vi "UHR-Fleezers Control (host) - 10.6.vi"() -> ()   [LabVIEW 2011] (continued)
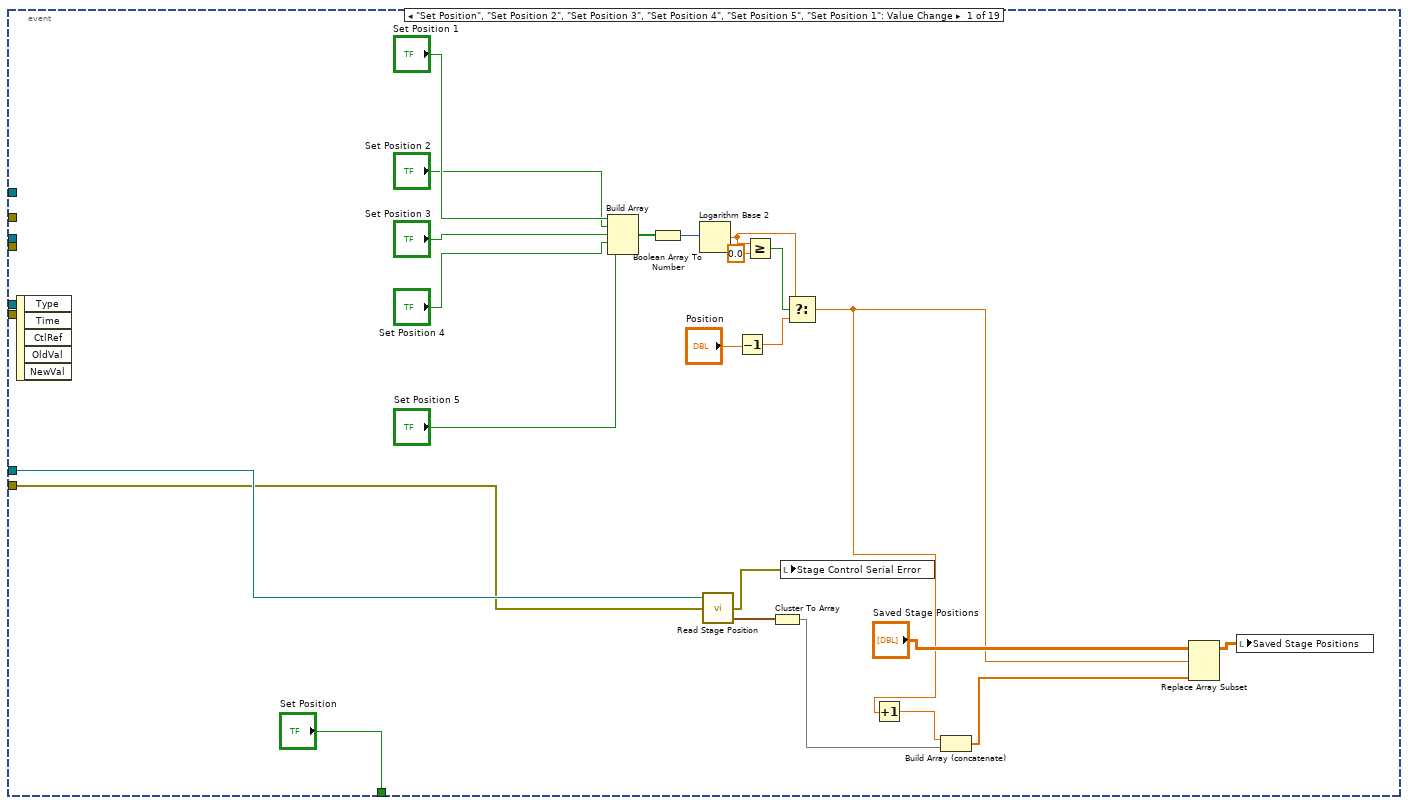
[diagram p2: hidden frame]
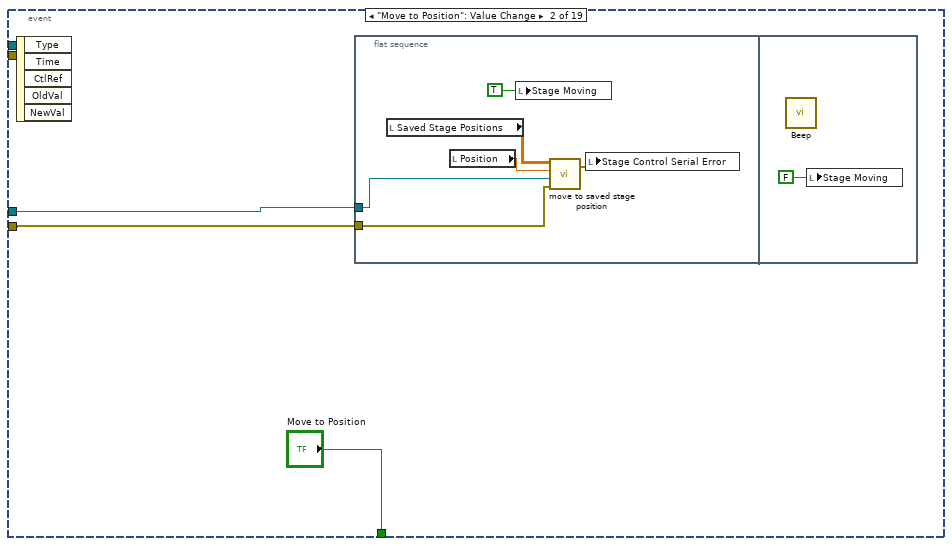
[diagram p3: hidden frame]
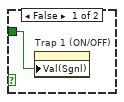
[diagram p5: hidden frame]
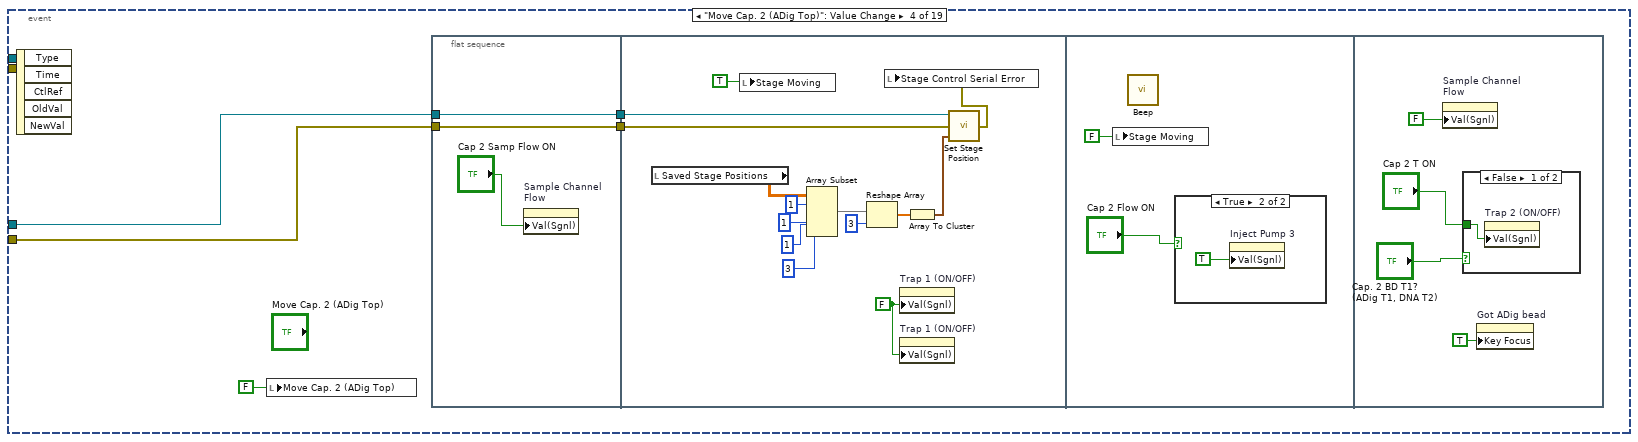
[diagram p6: hidden frame]
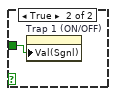
[diagram p8: hidden frame]
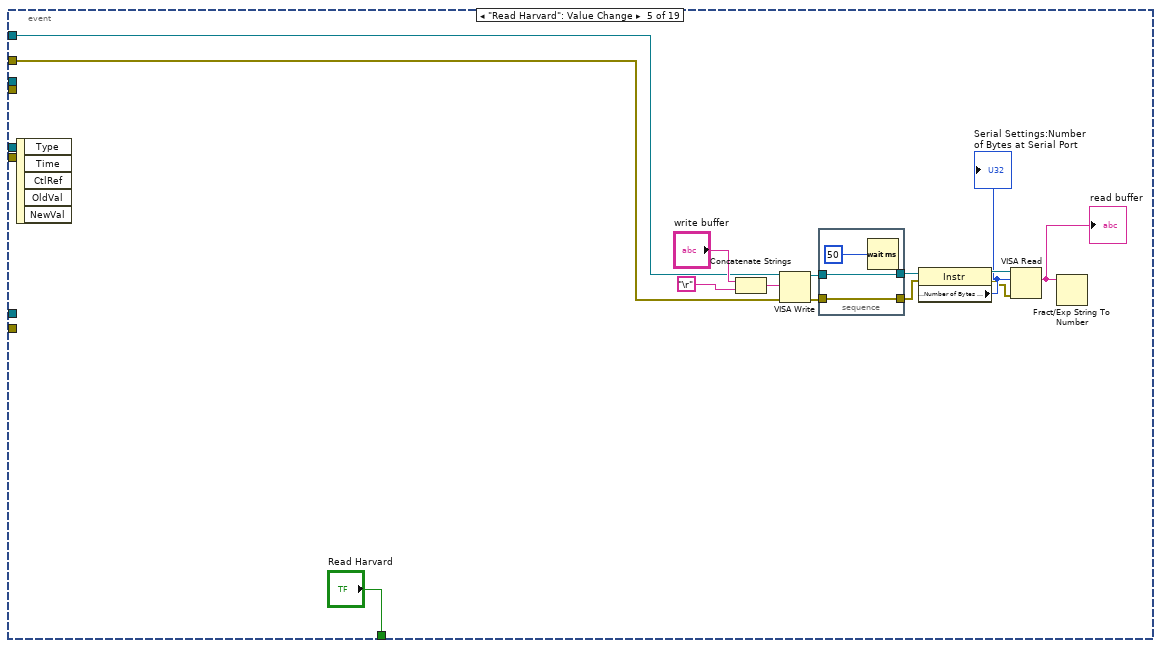
[diagram p9: hidden frame]
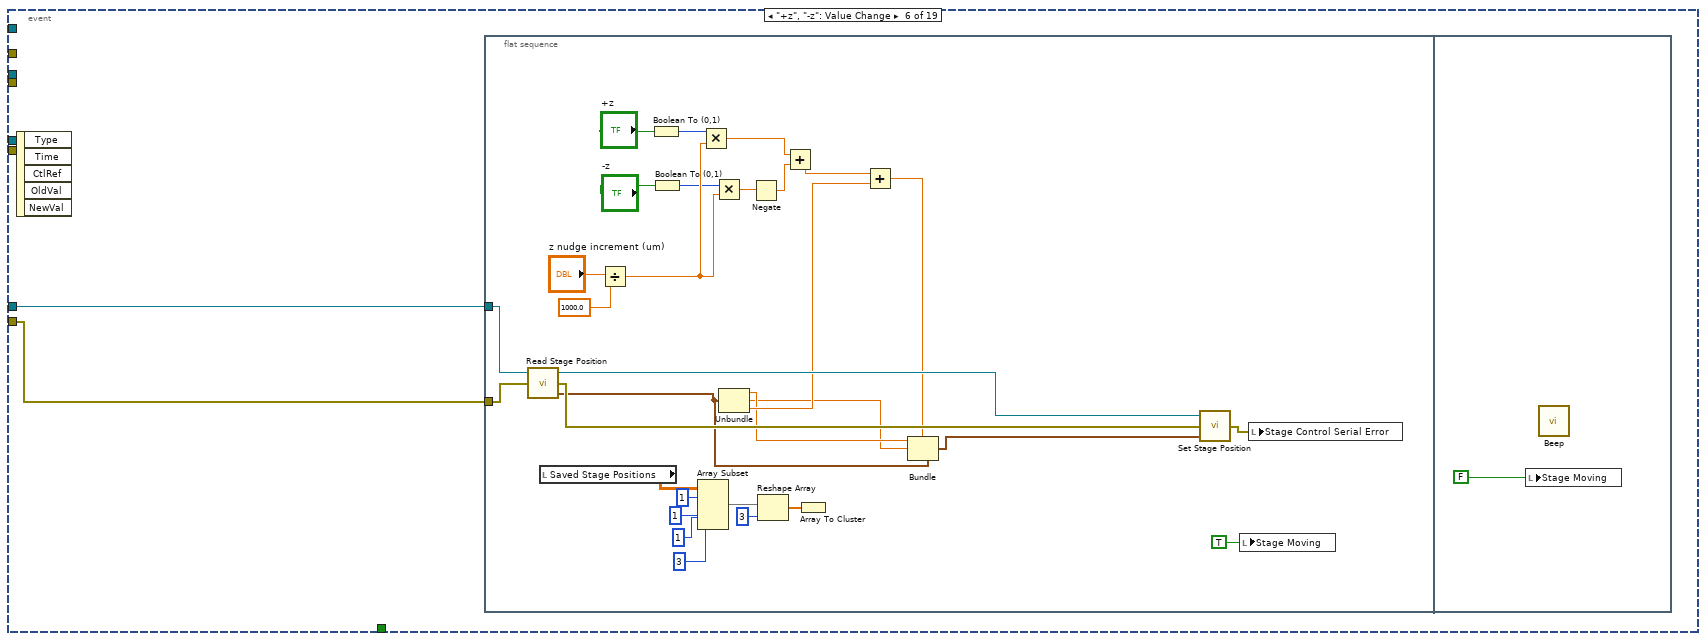
[diagram p10: hidden frame]
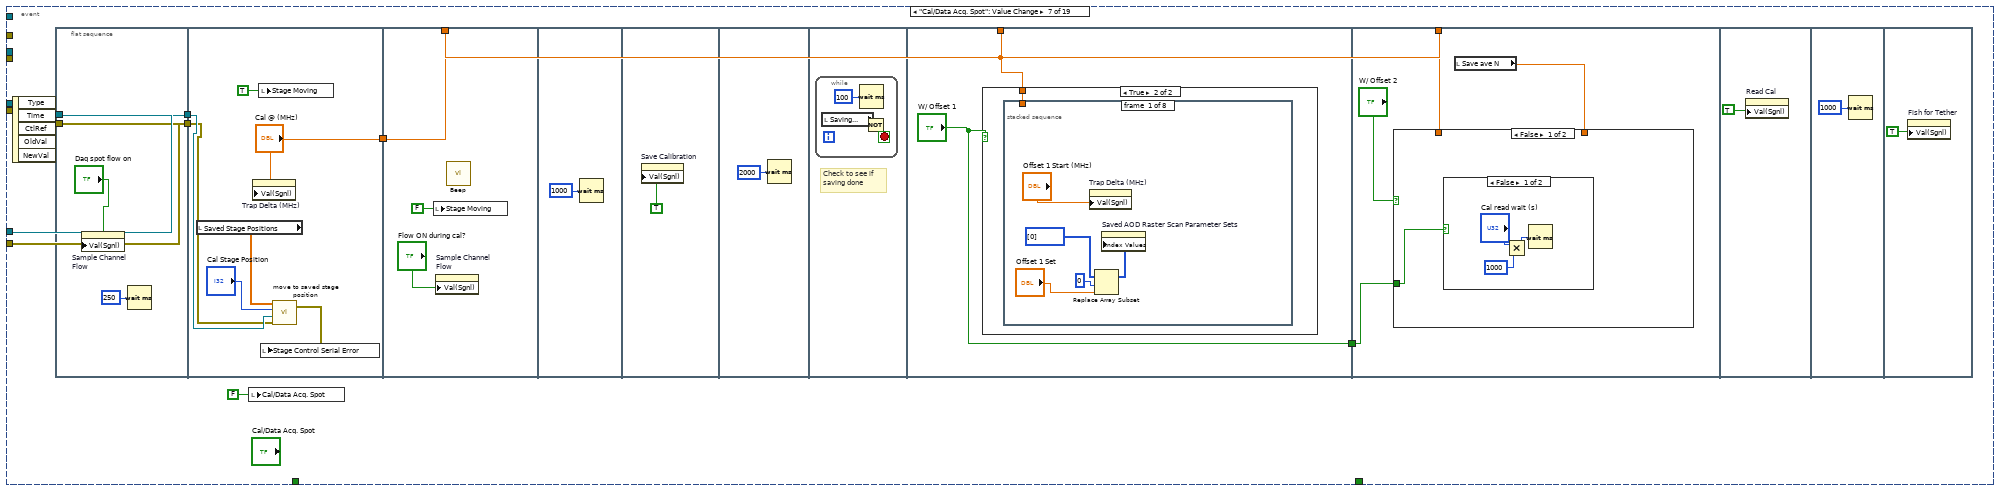
[diagram p11: hidden frame]
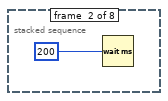
[diagram p13: hidden frame]
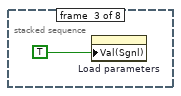
[diagram p14: hidden frame]
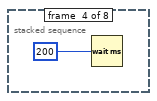
[diagram p15: hidden frame]
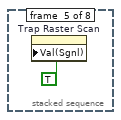
[diagram p16: hidden frame]
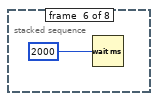
[diagram p17: hidden frame]
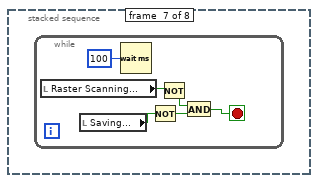
[diagram p18: hidden frame]
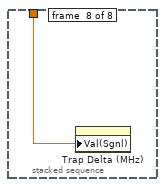
[diagram p19: hidden frame]
        w3951 = 32767.0 ("y")
        # "to return scan values\nafter a synchronous \nAOM scan"
        n2755 = local read "AO2"() -> (w3945:dbl)
        n2756 = local read "AO1"() -> (w3946:dbl)
        n2757 = local write "wait to reset values"(FALSE ("wait to reset values")) -> ()
        n2758 = Multiply(x=w3946, y=w3951) -> (x*y=w3948:dbl)
        n2759 = Multiply(x=w3945, y=w3951) -> (x*y=w3950:dbl)
        n2760 = Divide(x=w3948, y=w3952) -> (x/y=w3947:dbl)
        n2761 = Divide(x=w3950, y=w3952) -> (x/y=w3949:dbl)
        n2762 = To Word Integer(number=w3947) -> (16bit integer=w3953:i16)
        n2763 = To Word Integer(number=w3949) -> (16bit integer=w3954:i16)
        n2764 = local read "Total Counts (ticks)"() -> (w3938:u32)
        n2765 = xnode "Read/Write Control"("FPGA VI Reference In"=w3944, "error in"=w3942, "AO1"=w3953, "AO2"=w3954, "MCL count"=w3938) -> ("FPGA VI Reference Out"=w3943:T19, "error out"=w3941:errorcluster)
        n2766 = local read "Scan Range (V)\n(of steps)"() -> (w3939:dbl)
        n2767 = property on="Scan Range (V)\n(of steps)" class="DigNum (strict)"("Val(Sgnl)"=w3939) -> ()  [unwired: 2 in, 2 out]
      }
    }
    n2768 = node-c288() -> ()  [unwired: 2 out]
  }
  n2769 = node-c288(w91) -> ()  [unwired: 1 out]
  n2770 = node-c288(w93) -> ()  [unwired: 1 out]
  n2771 = node-c288(w78) -> ()  [unwired: 1 out]
  n2772 = VISA Close(VISA resource name=w82, error in (no error)=w81) -> (error out=w130:errorcluster)
  n2773 = call <vilib>:"Simple Error Handler.vi"("error in (no error)"=w130) -> ()  [unwired: 1 in, 8 out]
  n2774 = node-c288(w89) -> ()  [unwired: 1 out]
  n2775 = node-c288(w174) -> ()  [unwired: 1 out]
  n2776 = flat-sequence {
    tunnel: w268 -> [w4525]
    tunnel: w270 -> [w4526]
    tunnel: [w4524] -> w249
    tunnel: [w4523] -> w248
    tunnel: w230 -> [_]
    tunnel: w182 -> [_]
    tunnel: w95 -> [_]
    tunnel: w249 -> [w4527]
    tunnel: w248 -> [w4528]
    frame #0 {
      w4522 = FALSE ("AI to FIFO")
      n2777 = xnode "Read/Write Control"("FPGA VI Reference In"=w4526, "error in"=w4525, "AI to FIFO"=w4522, "APD to FIFO"=w4522) -> ("FPGA VI Reference Out"=w4524:T19, "error out"=w4523:errorcluster)
    }
    frame #1 {
      n2778 = xnode "Close FPGA VI Reference"("FPGA VI Reference In"=w4527, "error in"=w4528) -> ("error out"=→"error out":errorcluster)
    }
  }
